vi "_Validate Parameter.vi"(6 "Parameter":T1 {"Expt"."Mass Range"."Resolution Type" items=["High/High", "Medium/Medium", "Low/Low", "High/Medium", "High/Low", "Medium/High", "Medium/Low", "Low/High", "Low/Medium"]}, 9 "error in (no error)":errorcluster) -> (0 "Ch ID":i32[](array[numeric]), 1 "General Param":i32[](array[numeric]), 2 "RunMode":i32, 3 "error out":errorcluster, 4 "Low Values":i32[](array[numeric]), 5 "High Values (DAC)":i32[](array[numeric]))   [LabVIEW 2015]
uses:
  Type/_RT Parameter.ctl
  Type/_RT Active Ch.ctl
  Type/_RT Expt.ctl
  Type/_Run Mode.ctl
  Type/_RT Mass Range.ctl
  Type/_RT Res Type.ctl
  Type/_RT Instrument State.ctl
  _RT Global.vi
panel:
  # "General Parameters:\n===============\nRun Mode\n# of Ch's\nHigh Level Time (uS) / Q1 Pol\nLow Level Time (uS) / Q2 Pol"
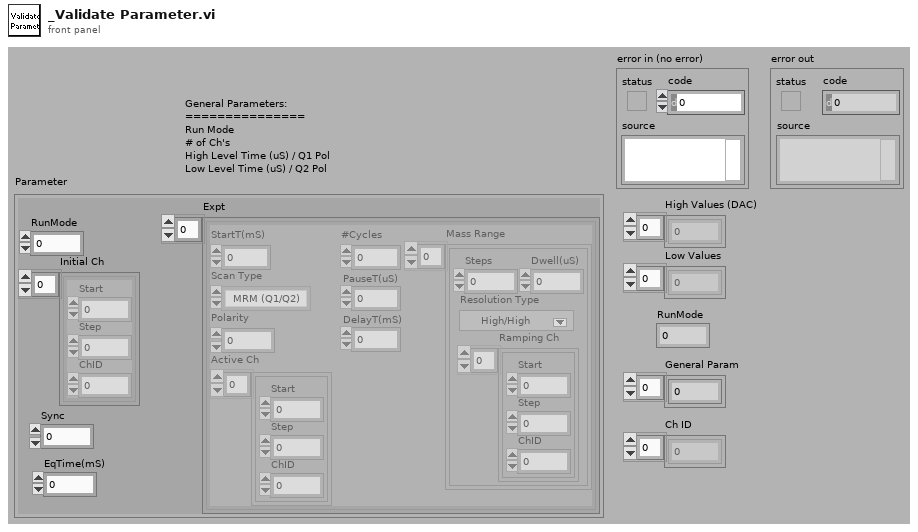
[diagram p1: front panel]
types:
  T1 = typedef "_RT Parameter.ctl" = cluster{"RunMode":i32, "Initial Ch":T2[], "Sync":u8, "Expt":T3[], "EqTime(mS)":i32}
  T2 = typedef "_RT Active Ch.ctl" = cluster{"Start":i32, "Step":i32, "ChID":i32}
  T3 = typedef "_RT Expt.ctl" = cluster{"StartT(mS)":i32, "#Cycles":i32, "Scan Type":T4, "PauseT(uS)":i32, "Polarity":u8, "DelayT(mS)":i32, "Active Ch":T2[], "Mass Range":T5[]}
  T4 = typedef "_Run Mode.ctl" = enum16{"MRM (Q1/Q2)", "Q1 Scan", "Q1 SRM", "Q2 Scan", "Q2 SRM", "Product Scan", "Precursor Scan", "Neutral Loss", "Neutral Gain"}
  T5 = typedef "_RT Mass Range.ctl" = cluster{"Steps":i32, "Dwell(uS)":i32, "Resolution Type":T6, "Ramping Ch":T2[]}
  T6 = typedef "_RT Res Type.ctl" = u16
  T7 = typedef "_RT Instrument State.ctl" = enum16{"Initializing", "Mass Spectrometer is Off", "Starting Up", "Turning Power Off", "Going to Standby", "Roughing Pump Ready", "Turning Turbo Off", "Turbo Startup", "Turbopump Ready", "Checking Vacuum", "Going to Ready", "Ready", "Running", "Source Standby", "Lost Communication", "Shutting Down", "Fault", "24V Standby", "Go to 24V Standby", "Turbopump Ready-Waiting"}
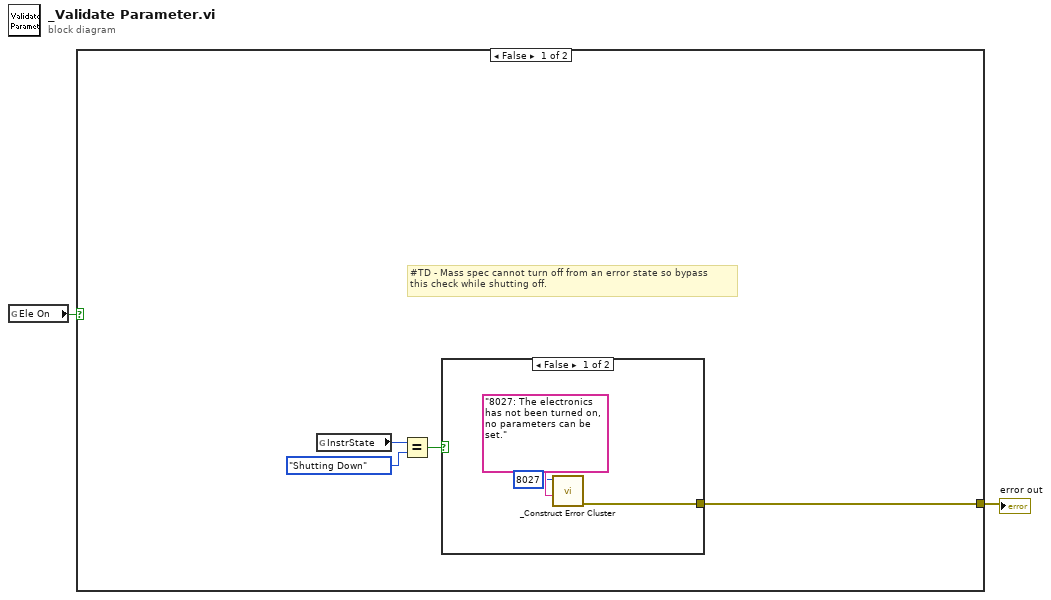
[diagram p0: block diagram]
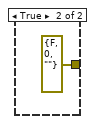
[diagram p2: hidden frame]
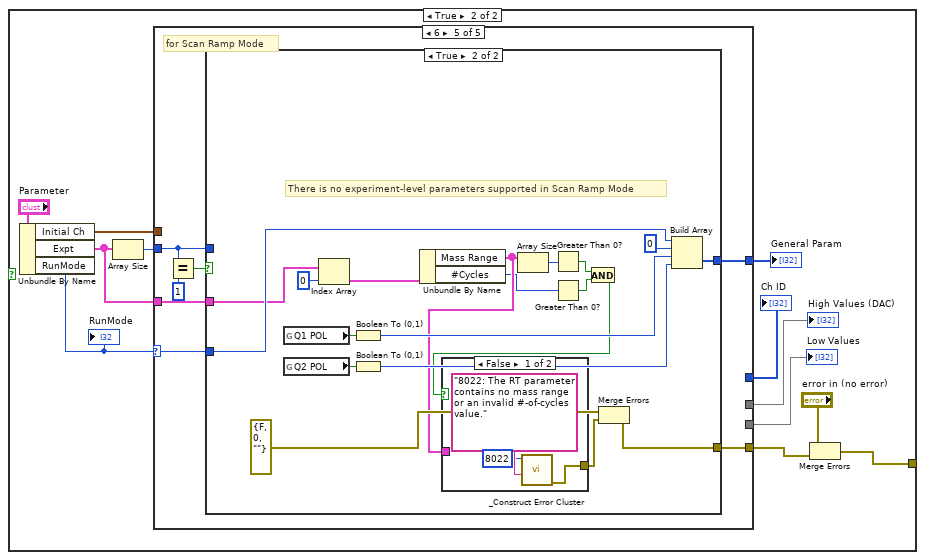
[diagram p3: hidden frame]
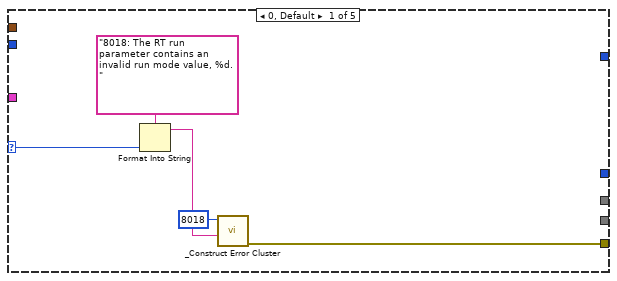
[diagram p4: hidden frame]
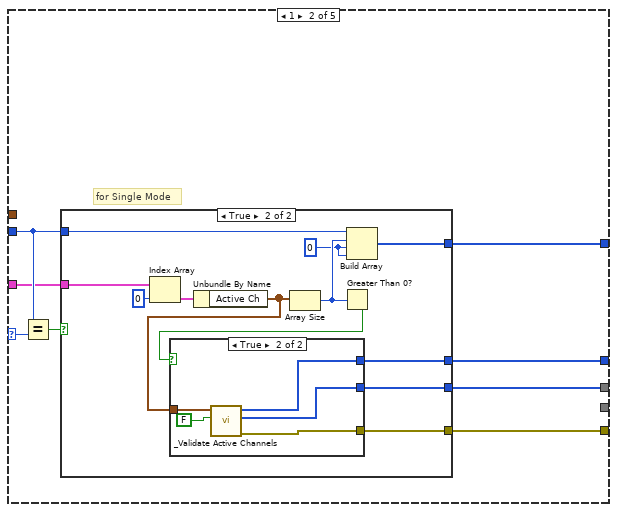
[diagram p5: hidden frame]
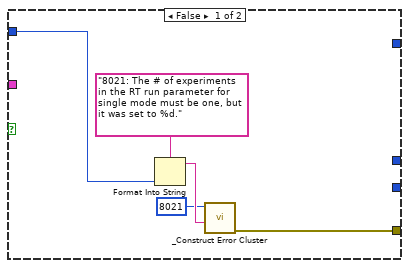
[diagram p6: hidden frame]
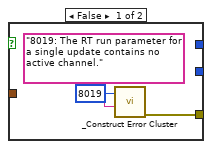
[diagram p7: hidden frame]
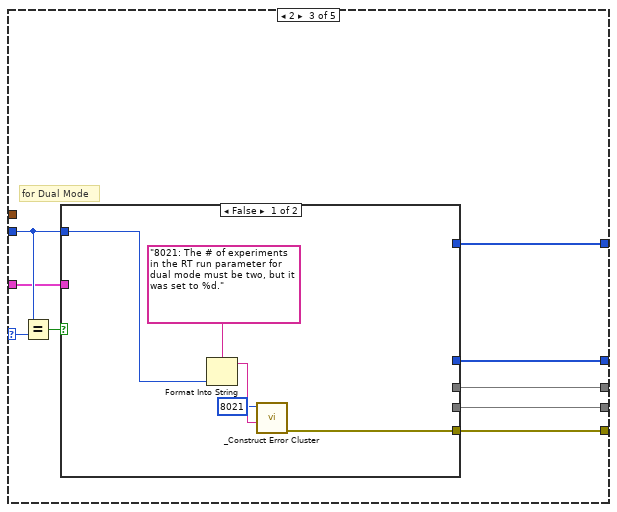
[diagram p8: hidden frame]
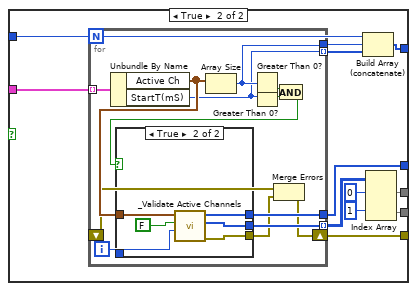
[diagram p9: hidden frame]
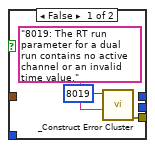
[diagram p10: hidden frame]
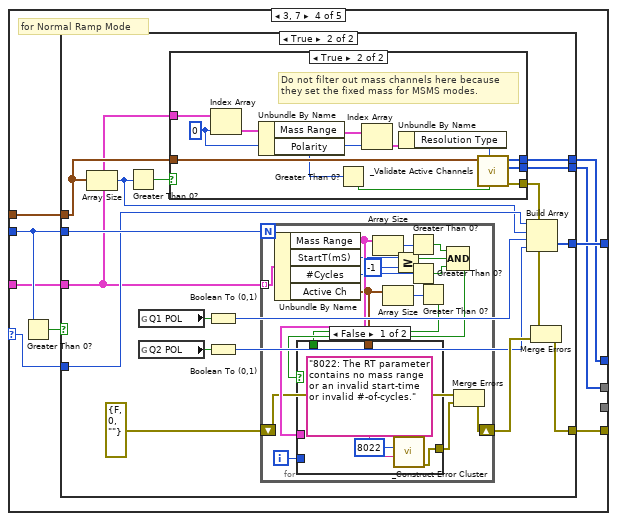
[diagram p11: hidden frame]
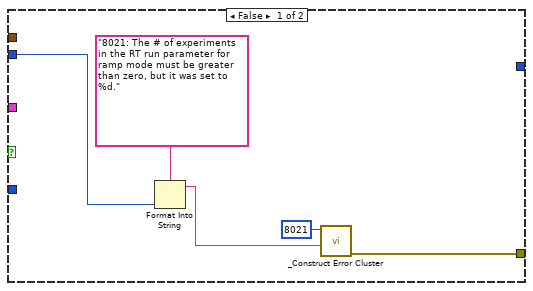
[diagram p12: hidden frame]
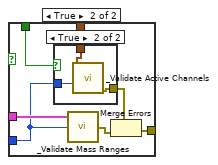
[diagram p14: hidden frame]
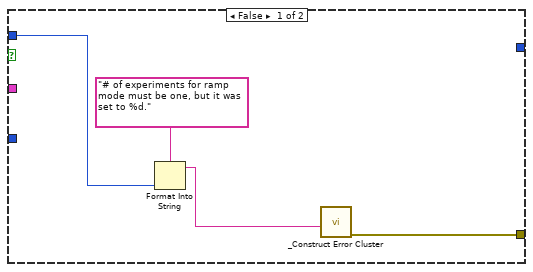
[diagram p16: hidden frame]
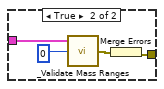
[diagram p17: hidden frame]
diagram:
  n1 = global read "_RT Global.vi" "Ele On"() -> (w1:bool)
  n2 = case shown="False" w1 {
    tunnel: [w6 w18] -> w2
    frame False {
      # "#TD - Mass spec cannot turn off from an error state so bypass\nthis check while shutting off."
      n3 = global read "_RT Global.vi" "InstrState"() -> (w5:T7)
      n4 = Equal?(x=w5, y=_RT_Instrument_State."Shutting Down") -> (x = y?=w3:bool)
      n5 = case shown="False" w3 {
        tunnel: [w9 errorcluster {"status"=FALSE, "code"=0, "source"=""} ("error out")] -> w6
        frame False {
          n6 = call "_Construct Error Cluster.vi"("reason"="8027: The electronics has not been turned on, no parameters can be set.", "errorCode"=8027) -> ("error out"=w9:errorcluster)  [unwired: 2 in, 3 out]
        }
        frame True {
        }
      }
    }
    frame True {
      n7 = Unbundle By Name("Parameter") -> ("Initial Ch"=w11:T2[], "Expt"=w22:T3[], "RunMode"=w12:i32)
      "RunMode" <- w12
      n8 = Array Size(array=w22) -> (size(s)=w21:i32)
      n9 = case shown="6" w12 {
        selector: w12 -> [w26 w33 w67 w109 w184]
        tunnel: [w25 w35 w69 w117 w188] -> w20
        tunnel: w22 -> [_ w31 w65 w114 w186]
        tunnel: w21 -> [_ w32 w66 w115 w183]
        tunnel: [_ w30 w63 w111 _] -> w17
        tunnel: [_ w29 w62 w110 _] -> w16
        tunnel: [_ w28 w64 w113 w185] -> w15
        tunnel: [_ _ w61 _ _] -> w14
        tunnel: w11 -> [_ _ _ w112 _]
        frame 0, Default {
          n10 = Format Into String(format string="8018: The RT run parameter contains an invalid run mode value, %d.", w26) -> (resulting string=w24:string)  [unwired: 2 in, 1 out]
          n11 = call "_Construct Error Cluster.vi"("reason"=w24, "errorCode"=8018) -> ("error out"=w25:errorcluster)  [unwired: 2 in, 3 out]
        }
        frame 1 {
          # "for Single Mode"
          n12 = Equal?(x=w32, y=w33) -> (x = y?=w34:bool)
          n13 = case shown="True" w34 {
            tunnel: [w40 w48] -> w35
            tunnel: w32 -> [w38 w44]
            tunnel: w31 -> [_ w52]
            tunnel: [_ w46] -> w30
            tunnel: [_ w45] -> w29
            tunnel: [_ w41] -> w28
            frame False {
              n14 = Format Into String(format string="8021: The # of experiments in the RT run parameter for single mode must be one, but it was set to %d.", w38) -> (resulting string=w37:string)  [unwired: 2 in, 1 out]
              n15 = call "_Construct Error Cluster.vi"("reason"=w37, "errorCode"=8021) -> ("error out"=w40:errorcluster)  [unwired: 2 in, 3 out]
            }
            frame True {
              w42 = 0 ("element")
              n16 = Index Array(array=w52, index=0) -> (element=w50:T3)
              n17 = Unbundle By Name(w50) -> ("Active Ch"=w47:T2[])
              n18 = Array Size(array=w47) -> (size(s)=w43:i32)
              n19 = Greater Than 0?(x=w43) -> (x > 0?=w49:bool)
              n20 = case shown="True" w49 {
                tunnel: [w54 w60] -> w48
                tunnel: w47 -> [_ w59]
                tunnel: [_ w58] -> w46
                tunnel: [_ w57] -> w45
                frame False {
                  n21 = call "_Construct Error Cluster.vi"("reason"="8019: The RT run parameter for a single update contains no active channel.", "errorCode"=8019) -> ("error out"=w54:errorcluster)  [unwired: 2 in, 3 out]
                }
                frame True {
                  n22 = call "_Validate Active Channels.vi"("User Res Table (T)"=FALSE, "Active Ch"=w59) -> ("error out"=w60:errorcluster, "DAC Values"=w57:i32[], "Ch ID"=w58:i32[])  [unwired: 4 in, 1 out]
                }
              }
              n23 = Build Array(w44, w43, w42, w42) -> (w41:i32[])
            }
          }
        }
        frame 2 {
          # "for Dual Mode"
          n24 = Equal?(x=w66, y=w67) -> (x = y?=w68:bool)
          n25 = case shown="False" w68 {
            tunnel: [w74 w86] -> w69
            tunnel: w66 -> [w72 w83]
            tunnel: w65 -> [_ w85]
            tunnel: [_ w84] -> w64
            tunnel: [_ w80] -> w63
            tunnel: [_ w76] -> w62
            tunnel: [_ w75] -> w61
            frame False {
              n26 = Format Into String(format string="8021: The # of experiments in the RT run parameter for dual mode must be two, but it was set to %d.", w72) -> (resulting string=w71:string)  [unwired: 2 in, 1 out]
              n27 = call "_Construct Error Cluster.vi"("reason"=w71, "errorCode"=8021) -> ("error out"=w74:errorcluster)  [unwired: 2 in, 3 out]
            }
            frame True {
              n28 = for {
                N: w83 -> [_]
                tunnel: w85 -> [w98] mode=indexing
                tunnel: [w94] -> w82
                tunnel: [w93] -> w81 mode=indexing
                tunnel: [w92] -> w80
                tunnel: [w91] -> w79 mode=indexing
                shift-right: [w89] -> w86
                shift-left: _ -> [w88]
                i -> [w87]
                n29 = Unbundle By Name(w98) -> ("Active Ch"=w99:T2[], "StartT(mS)"=w93:i32)
                n30 = Array Size(array=w99) -> (size(s)=w94:i32)
                n31 = Greater Than 0?(x=w94) -> (x > 0?=w96:bool)
                n32 = Greater Than 0?(x=w93) -> (x > 0?=w97:bool)
                n33 = And(x=w96, y=w97) -> (x .and. y?=w95:bool)
                n34 = case shown="True" w95 {
                  tunnel: [w101 w108] -> w90
                  tunnel: w99 -> [_ w107]
                  tunnel: [_ w106] -> w92
                  tunnel: [_ w105] -> w91
                  tunnel: w87 -> [_ w103]
                  frame False {
                    n35 = call "_Construct Error Cluster.vi"("reason"="8019: The RT run parameter for a dual run contains no active channel or an invalid time value.", "errorCode"=8019) -> ("error out"=w101:errorcluster)  [unwired: 2 in, 3 out]
                  }
                  frame True {
                    n36 = call "_Validate Active Channels.vi"("Expt#"=w103, "User Res Table (T)"=FALSE, "Active Ch"=w107) -> ("error out"=w108:errorcluster, "DAC Values"=w105:i32[], "Ch ID"=w106:i32[])  [unwired: 3 in, 1 out]
                  }
                }
                n37 = Merge Errors(w88, w90) -> (w89:errorcluster)
              }
              n38 = Build Array (concatenate)(w83, w82, w81) -> (w84:i32[])
              n39 = Index Array(array=w79, index (row) #1=0 ("index (row)"), index (row) #2=1 ("index (row)")) -> (element #1=w76:i32[], element #2=w75:i32[])  [unwired: 2 in]
            }
          }
        }
        frame 3, 7 {
          # "for Normal Ramp Mode"
          n40 = Greater Than 0?(x=w115) -> (x > 0?=w116:bool)
          n41 = case shown="True" w116 {
            tunnel: [w122 w133] -> w117
            tunnel: w115 -> [w120 w139]
            tunnel: w114 -> [_ w127]
            tunnel: [_ w138] -> w113
            tunnel: w112 -> [_ w136]
            tunnel: [_ w132] -> w111
            tunnel: [_ w131] -> w110
            tunnel: w109 -> [_ w129]
            frame False {
              n42 = Format Into String(format string="8021: The # of experiments in the RT run parameter for ramp mode must be greater than zero, but it was set to %d.", w120) -> (resulting string=w119:string)  [unwired: 2 in, 1 out]
              n43 = call "_Construct Error Cluster.vi"("reason"=w119, "errorCode"=8021) -> ("error out"=w122:errorcluster)  [unwired: 2 in, 3 out]
            }
            frame True {
              n44 = Array Size(array=w136) -> (size(s)=w128:i32)
              n45 = Greater Than 0?(x=w128) -> (x > 0?=w137:bool)
              n46 = global read "_RT Global.vi" "Q1 POL"() -> (w125:bool)
              n47 = global read "_RT Global.vi" "Q2 POL"() -> (w126:bool)
              n48 = case shown="True" w137 {
                tunnel: [_ w151] -> w135
                tunnel: w136 -> [_ w148]
                tunnel: [_ w150] -> w132
                tunnel: [_ w149] -> w131
                tunnel: w127 -> [_ w147]
                frame False {
                }
                frame True {
                  w142 = 0 ("index")
                  # "Do not filter out mass channels here because\nthey set the fixed mass for MSMS modes."
                  n49 = Index Array(array=w147, index=w142) -> (element=w146:T3)
                  n50 = Unbundle By Name(w146) -> ("Mass Range"=w145:T5[], "Polarity"=w141:u8)
                  n51 = Greater Than 0?(x=w141) -> (x > 0?=w140:bool)
                  n52 = Index Array(array=w145, index=w142) -> (element=w144:T5)
                  n53 = Unbundle By Name(w144) -> ("Resolution Type"=w143:T6)
                  n54 = call "_Validate Active Channels.vi"("Negative (F)"=w140, "Resolution Type"=w143, "Active Ch"=w148) -> ("error out"=w151:errorcluster, "DAC Values"=w149:i32[], "Ch ID"=w150:i32[])  [unwired: 3 in, 1 out]
                }
              }
              n55 = Boolean To (0,1)(Boolean=w125) -> (0, 1=w124:i16)
              n56 = Boolean To (0,1)(Boolean=w126) -> (0, 1=w123:i16)
              n57 = for {
                N: w139 -> [_]
                tunnel: w127 -> [w166] mode=indexing
                shift-right: [w157] -> w134
                shift-left: errorcluster {"status"=FALSE, "code"=0, "source"=""} ("error out") -> [w156]
                i -> [w155]
                n58 = Unbundle By Name(w166) -> ("Mass Range"=w167:T5[], "StartT(mS)"=w153:i32, "#Cycles"=w163:i32, "Active Ch"=w159:T2[])
                n59 = Array Size(array=w167) -> (size(s)=w168:i32)
                n60 = Array Size(array=w159) -> (size(s)=w161:i32)
                n61 = Greater Or Equal?(x=w153, y=-1) -> (x >= y?=w154:bool)
                n62 = Greater Than 0?(x=w168) -> (x > 0?=w165:bool)
                n63 = Greater Than 0?(x=w163) -> (x > 0?=w162:bool)
                n64 = Greater Than 0?(x=w161) -> (x > 0?=w160:bool)
                n65 = Compound Arithmetic op=AND(w165, w154, w162) -> (w164:bool)
                n66 = case shown="False" w164 {
                  tunnel: [w170 w175] -> w158
                  tunnel: w167 -> [_ w176]
                  tunnel: w160 -> [_ w178]
                  tunnel: w159 -> [_ w177]
                  tunnel: w155 -> [_ w172]
                  frame False {
                    n67 = call "_Construct Error Cluster.vi"("reason"="8022: The RT parameter contains no mass range or an invalid start-time or invalid #-of-cycles.", "errorCode"=8022) -> ("error out"=w170:errorcluster)  [unwired: 2 in, 3 out]
                  }
                  frame True {
                    n68 = case shown="True" w178 {
                      tunnel: w177 -> [_ w181]
                      tunnel: [_ w180] -> w174
                      tunnel: w172 -> [_ w179]
                      frame False {
                      }
                      frame True {
                        n69 = call "_Validate Active Channels.vi"("Expt#"=w179, "Active Ch"=w181) -> ("error out"=w180:errorcluster)  [unwired: 4 in, 3 out]
                      }
                    }
                    n70 = call "_Validate Mass Ranges.vi"("Expt#"=w172, "Mass Range"=w176) -> ("error out"=w173:errorcluster)  [unwired: 1 in]
                    n71 = Merge Errors(w174, w173) -> (w175:errorcluster)
                  }
                }
                n72 = Merge Errors(w156, w158) -> (w157:errorcluster)
              }
              n73 = Build Array(w129, w128, w124, w123) -> (w138:i32[])
              n74 = Merge Errors(w135, w134) -> (w133:errorcluster)
            }
          }
        }
        frame 6 {
          # "for Scan Ramp Mode"
          n75 = Equal?(x=w183, y=1) -> (x = y?=w187:bool)
          n76 = case shown="True" w187 {
            tunnel: [w192 w203] -> w188
            tunnel: w183 -> [w190 _]
            tunnel: w186 -> [_ w195]
            tunnel: [_ w211] -> w185
            tunnel: w184 -> [_ w209]
            frame False {
              n77 = Format Into String(format string="# of experiments for ramp mode must be one, but it was set to %d.", w190) -> (resulting string=w189:string)  [unwired: 2 in, 1 out]
              n78 = call "_Construct Error Cluster.vi"("reason"=w189) -> ("error out"=w192:errorcluster)  [unwired: 3 in, 3 out]
            }
            frame True {
              # "There is no experiment-level parameters supported in Scan Ramp Mode"
              n79 = global read "_RT Global.vi" "Q1 POL"() -> (w207:bool)
              n80 = global read "_RT Global.vi" "Q2 POL"() -> (w208:bool)
              n81 = Index Array(array=w195, index=0) -> (element=w193:T3)
              n82 = Boolean To (0,1)(Boolean=w207) -> (0, 1=w206:i16)
              n83 = Boolean To (0,1)(Boolean=w208) -> (0, 1=w205:i16)
              n84 = Unbundle By Name(w193) -> ("Mass Range"=w201:T5[], "#Cycles"=w198:i32)
              n85 = Array Size(array=w201) -> (size(s)=w202:i32)
              n86 = Greater Than 0?(x=w202) -> (x > 0?=w200:bool)
              n87 = Greater Than 0?(x=w198) -> (x > 0?=w197:bool)
              n88 = And(x=w200, y=w197) -> (x .and. y?=w199:bool)
              n89 = case shown="False" w199 {
                tunnel: [w213 w217] -> w196
                tunnel: w201 -> [_ w218]
                frame False {
                  n90 = call "_Construct Error Cluster.vi"("reason"="8022: The RT parameter contains no mass range or an invalid #-of-cycles value.", "errorCode"=8022) -> ("error out"=w213:errorcluster)  [unwired: 2 in, 3 out]
                }
                frame True {
                  n91 = call "_Validate Mass Ranges.vi"("Expt#"=0, "Mass Range"=w218) -> ("error out"=w216:errorcluster)  [unwired: 1 in]
                  n92 = Merge Errors(w216) -> (w217:errorcluster)
                }
              }
              n93 = Merge Errors(errorcluster {"status"=FALSE, "code"=0, "source"=""} ("error out"), w196) -> (w203:errorcluster)
              n94 = Build Array(w209, 0 ("size(s)"), w206, w205) -> (w211:i32[])
            }
          }
        }
      }
      "General Param" <- w15
      "Ch ID" <- w17
      "High Values (DAC)" <- w16
      "Low Values" <- w14
      n95 = Merge Errors("error in (no error)", w20) -> (w18:errorcluster)
    }
  }
  "error out" <- w2
